vi "Read Controller Message Type.vi"(8 "error in (no error)":errorcluster, 11 "Controller Message in":refnum<class "Controller Message.lvclass">) -> (0 "error out":errorcluster, 2 "Controller Message Type":T1, 3 "Controller Message out":refnum<class "Controller Message.lvclass">)   [LabVIEW 2015, in "RDS Child Messages.lvlib" / "Controller Message.lvclass"]
uses:
  Controller Message.lvclass
  Controller Message Type.ctl
  Controller Message.lvclass/Controller Message.ctl
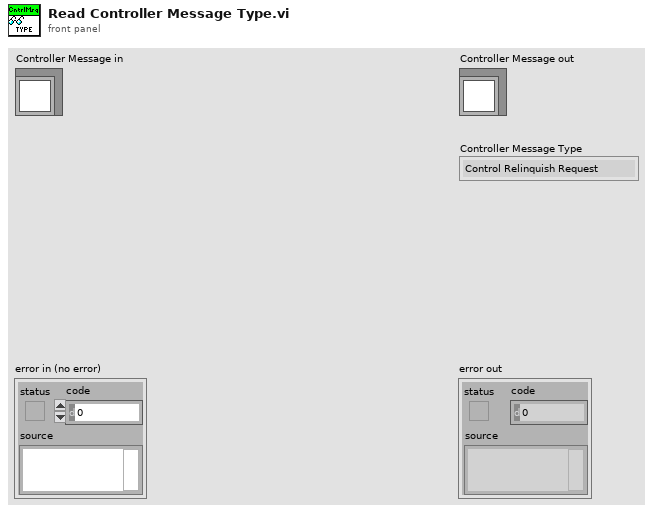
[diagram p1: front panel]
types:
  T1 = typedef "RDS Child Messages.lvlib/Controller Message.lvclass/Controller Message Type.ctl" = enum16{"Control Relinquish Request", "Control Relinquish Command", "Control Request", "Control Granted"}
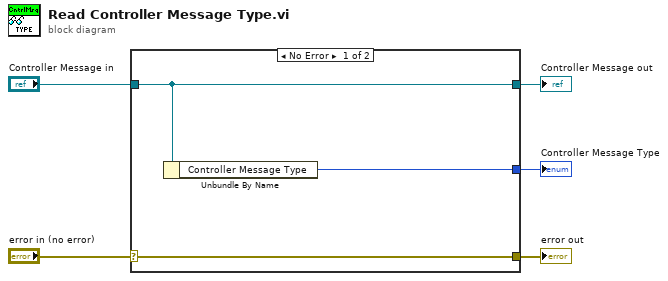
[diagram p0: block diagram]
diagram:
  n1 = case shown="No Error" "error in (no error)" {
    selector: "error in (no error)" -> [w8 w9]
    tunnel: [w8 w9] -> w4
    tunnel: [w7 w10] -> w2
    tunnel: "Controller Message in" -> [w7 w10]
    tunnel: [w6 _] -> w1
    frame No Error {
      n2 = Unbundle By Name(w7) -> ("Controller Message Type"=w6:T1)
    }
    frame Error {
    }
  }
  "error out" <- w4
  "Controller Message out" <- w2
  "Controller Message Type" <- w1
